vi "Send.vi"(6 "# Retires (1)":i32=1, 7 "Pump ID (0:A)":T1, 8 "error in (no error)":errorcluster, 10 "Command":string, 11 "VISA resource in":refnum<visa-resource-name>) -> (0 "error out":errorcluster, 2 "Information":string, 3 "VISA resource out":refnum<visa-resource-name>)   [LabVIEW 2020, in "Global FIA milliGAT.lvlib"]
doc: "Sends a command to the motor controller and receives a response back. The response is parsed for confirmation that the intended message was received by the controller, that the message was valid, and for any information prompted for by the message."
uses:
  <instrlib>/RxnRover/Global FIA milliGAT 3.14/Global FIA milliGAT.lvlib
  <instrlib>/RxnRover/Global FIA milliGAT 3.14/Public/Utility/Pump Address.ctl
  <vilib>/Utility/error.llb/DialogType.ctl
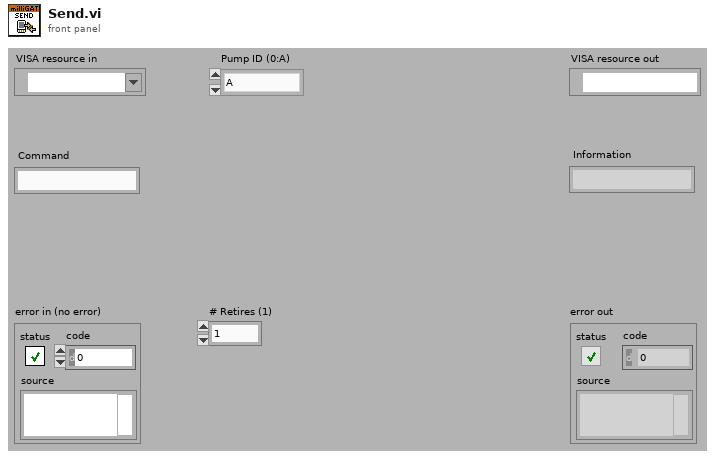
[diagram p1: front panel]
types:
  T1 = typedef "Global FIA milliGAT.lvlib/Pump Address.ctl" = enum16{"A", "B", "C", "D", "E", "F", "G", "H", "I", "J", "K", "L", "M", "N", "O", "P", "Q", "R", "S", "T", "U", "V", "W", "X", "Y", "Z", "a", "b", "c", "d", "e", "f", "g", "h", "i", "j", "k", "l", "m", "n", "o", "p", "q", "r", "s", "t", "u", "v", "w", "x", "y", "z", "0", "1", "2", "3", "4", "5", "6", "7", "8", "9"}
  T2 = typedef "Semaphore RefNum" = refnum<k1>
  T3 = typedef "DialogType.ctl" = u16
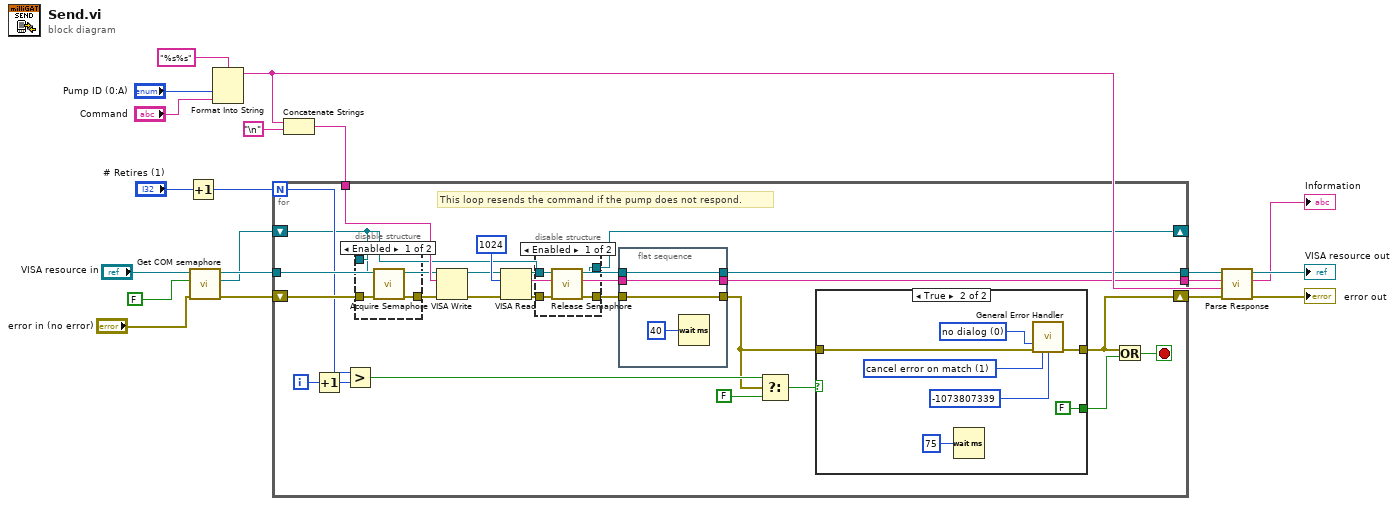
[diagram p0: block diagram]
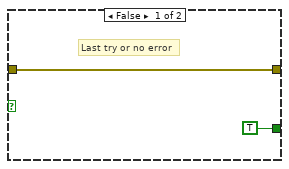
[diagram p4: hidden frame]
diagram:
  n1 = Increment(x="# Retires (1)") -> (x+1=w13:i32)
  n2 = call <instrlib>:"Get COM semaphore.vi"("error in (no error)"="error in (no error)", "create if not found (T)"=FALSE, "VISA resource in"="VISA resource in") -> ("error out"=w4:errorcluster, "semaphore"=w2:T2, "VISA resource out"=w3:refnum<visa-resource-name>)  [unwired: 6 in]
  n3 = Format Into String(format string="%s%s", "Pump ID (0:A)", "Command") -> (resulting string=w8:string)  [unwired: 2 in, 1 out]
  n4 = Concatenate Strings(w8, "\n") -> (w19:string)
  n5 = for {
    N: w13 -> [w39]
    tunnel: w19 -> [w45]
    tunnel: [w26] -> w15
    shift-right: [w38] -> w11
    shift-left: w4 -> [w43]
    tunnel: [w28] -> w12
    tunnel: w3 -> [w42]
    shift-right: [w21] -> _
    shift-left: w2 -> [w22]
    i -> [w41]
    stop <- w36 stop-if-true
    # "This loop resends the command if the pump does not respond."
    n6 = Increment(x=w41) -> (x+1=w40:i32)
    n7 = Greater?(x=w39, y=w40) -> (0:w34:bool)
    n8 = disable-structure shown="Enabled" {
      disable-tunnel: w43 -> [w53 w54]
      disable-tunnel: [w52 w54] -> w24
      disable-tunnel: w22 -> [w51 _]
      frame Enabled {
        n9 = call <vilib>:"Acquire Semaphore.vi"("error in (no error)"=w53, "semaphore"=w51) -> ("error out"=w52:errorcluster)  [unwired: 3 in, 2 out]
      }
      frame Disabled {
      }
    }
    n10 = VISA Write(VISA resource name=w42, write buffer=w45, error in (no error)=w24) -> (VISA resource name out=w32:refnum<visa-resource-name>, error out=w31:errorcluster)  [unwired: 1 out]
    n11 = VISA Read(VISA resource name=w32, byte count=u32 1024, error in (no error)=w31) -> (VISA resource name out=w30:refnum<visa-resource-name>, read buffer=w27:string, error out=w29:errorcluster)  [unwired: 1 out]
    n12 = disable-structure shown="Enabled" {
      disable-tunnel: w29 -> [w49 w50]
      disable-tunnel: [w48 w50] -> w23
      disable-tunnel: w22 -> [w47 _]
      disable-tunnel: [w46 _] -> w21
      frame Enabled {
        n13 = call <vilib>:"Release Semaphore.vi"("error in (no error)"=w49, "semaphore"=w47) -> ("error out"=w48:errorcluster, "semaphore out"=w46:T2)  [unwired: 4 in]
      }
      frame Disabled {
      }
    }
    n14 = flat-sequence {
      tunnel: w30 -> [w56]
      tunnel: w23 -> [w57]
      tunnel: [w57] -> w25
      tunnel: [w56] -> w28
      tunnel: w27 -> [w55]
      tunnel: [w55] -> w26
      frame #0 {
        n15 = Wait (ms)(milliseconds to wait=u32 40) -> ()  [unwired: 1 out]
      }
    }
    n16 = Select(t=w34, s=w25, f=FALSE) -> (s? t:f=w33:bool)
    n17 = case shown="True" w33 {
      tunnel: w25 -> [w59 w67]
      tunnel: [w59 w66] -> w38
      tunnel: [TRUE FALSE] -> w37
      frame False {
        # "Last try or no error"
      }
      frame True {
        w64 = T3 0 items=["no dialog", "OK message", "continue or stop message", "OK message + warnings", "continue/stop + warnings"] ("type of dialog (OK msg:1)")
        w65 = 1 items=["no exception", "cancel error on match", "set error on match"] ("[exception action] (none:0)")
        n18 = Wait (ms)(milliseconds to wait=u32 75) -> ()  [unwired: 1 out]
        n19 = call <vilib>:"General Error Handler.vi"("type of dialog (OK msg:1)"=w64, "error in (no error)"=w67, "[exception action] (none:0)"=w65, "[exception code]"=-1073807339 ("[error code] (0)")) -> ("error out"=w66:errorcluster)  [unwired: 7 in, 4 out]
      }
    }
    n20 = Or(x=w38, y=w37) -> (x .or. y?=w36:bool)
  }
  n21 = call <instrlib>:"Parse Response.vi"("error in (no error)"=w11, "Command"=w8, "Response"=w15, "VISA resource in"=w12) -> ("error out"=→"error out":errorcluster, "Information"=→"Information":string, "VISA resource out"=→"VISA resource out":refnum<visa-resource-name>)  [unwired: 5 in]
